vi "QuickDrop Populate QDKS Listbox.vi"(4 "Listbox Value":i32 caption="列表框值", 5 "Plugin Path":refnum<vi> caption="插件路径", 6 "Plugin Description String":refnum<vi> caption="插件说明字符串", 7 "QDKS Info":T1[](array[typedef]) caption="QDKS信息", 9 "Set Shortcut Boolean":refnum<vi> caption="设置快捷方式布尔", 10 "Shortcut String":refnum<vi> caption="快捷键字符串", 11 "Mappings Listbox":refnum<vi> caption="映射列表框") -> (0 "No Desc out":string="（无说明信息）" caption="无说明输出", 1 "Default out":string="%s（默认）" caption="默认输出", 2 "Control out":string="Ctrl-%s" caption="Ctrl组合输出")   [LabVIEW 2016]
uses:
  <resource>/dialog/QuickDrop/QuickDrop QDKS Info.ctl
panel:
  in  "No Desc":string="（无说明信息）" caption="无说明"
  in  "Control":string="Ctrl-%s" caption="Ctrl组合"
  in  "Default":string="%s（默认）" caption="默认"
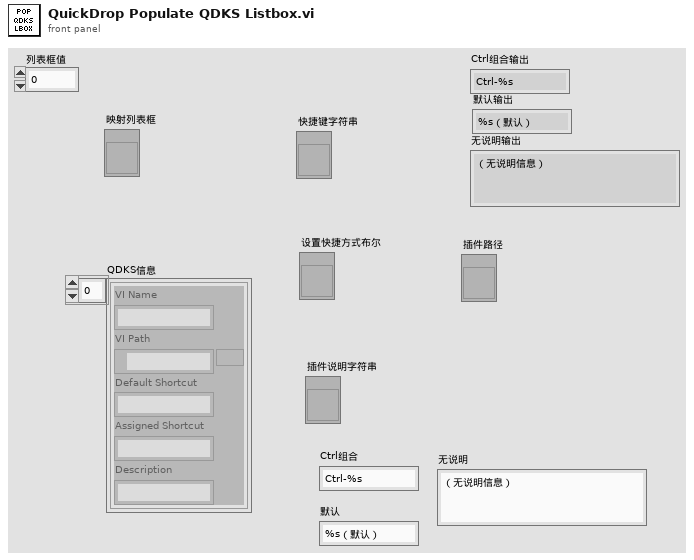
[diagram p1: front panel]
types:
  T1 = typedef "QuickDrop QDKS Info.ctl" = cluster{"VI Name":string, "VI Path":path, "Default Shortcut":string, "Assigned Shortcut":string, "Description":string}
  T2 = enum8{"Enabled", "Disabled", "Disabled and Grayed Out"}
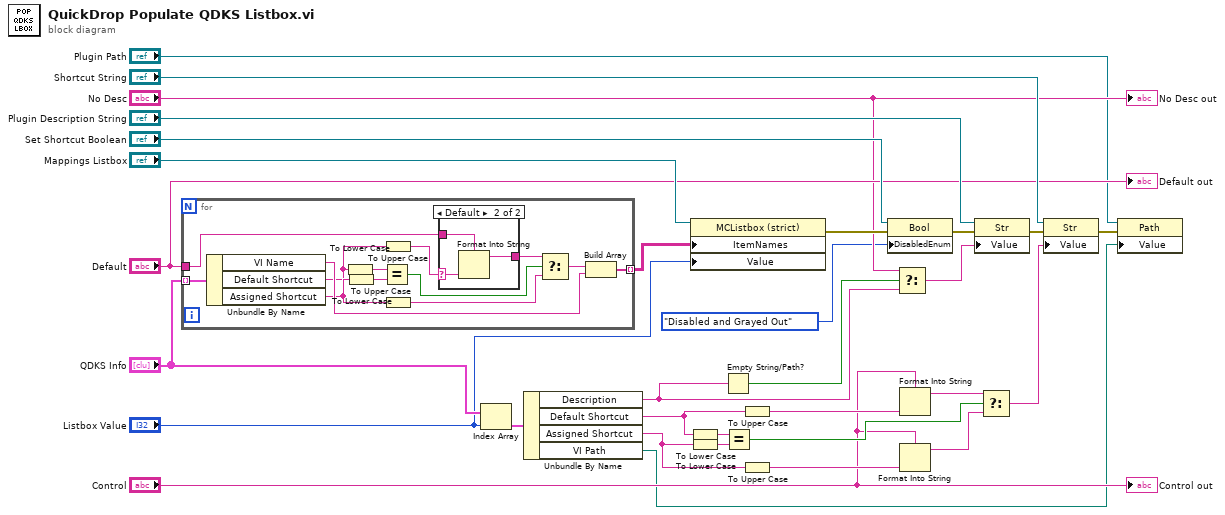
[diagram p0: block diagram]
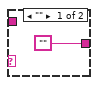
[diagram p2: hidden frame]
diagram:
  n1 = for {
    tunnel: "QDKS Info" -> [w44] mode=indexing
    tunnel: "Default" -> [w38]
    tunnel: [w32] -> w1 mode=indexing
    n2 = Unbundle By Name(w44) -> ("VI Name"=w43:string, "Default Shortcut"=w37:string, "Assigned Shortcut"=w41:string)
    n3 = To Lower Case(string=w37) -> (all lower case string=w34:string)
    n4 = To Lower Case(string=w41) -> (all lower case string=w33:string)
    n5 = Equal?(x=w34, y=w33) -> (x = y?=w42:bool)
    n6 = To Upper Case(1:w37) -> (0:w35:string)
    n7 = To Upper Case(1:w41) -> (0:w39:string)
    n8 = case shown="Default" w35 {
      selector: w35 -> [_ w46]
      tunnel: w38 -> [_ w48]
      tunnel: ["" w47] -> w36
      frame "" {
      }
      frame Default {
        n9 = Format Into String(format string=w48, w46) -> (resulting string=w47:string)  [unwired: 2 in, 1 out]
      }
    }
    n10 = Select(t=w36, s=w42, f=w39) -> (s? t:f=w40:string)
    n11 = Build Array(w40, w43) -> (w32:string[])
  }
  n12 = Index Array(array="QDKS Info", index="Listbox Value") -> (element=w25:T1)
  n13 = Unbundle By Name(w25) -> ("Description"=w14:string, "Default Shortcut"=w19:string, "Assigned Shortcut"=w23:string, "VI Path"=w2:path)
  n14 = To Lower Case(string=w19) -> (all lower case string=w7:string)
  n15 = To Lower Case(string=w23) -> (all lower case string=w6:string)
  n16 = property class="MCListbox (strict)"(reference="Mappings Listbox", "ItemNames"=w1, "Value"="Listbox Value") -> (error out=w30:errorcluster)  [unwired: 1 in, 1 out]
  n17 = Empty String/Path?(string/path=w14) -> (empty?=w15:bool)
  n18 = Equal?(x=w7, y=w6) -> (x = y?=w24:bool)
  n19 = To Upper Case(1:w19) -> (0:w17:string)
  n20 = To Upper Case(1:w23) -> (0:w10:string)
  n21 = property class="Bool"(reference="Set Shortcut Boolean", error in=w30, "DisabledEnum"=T2."Disabled and Grayed Out" ("Disabled")) -> (error out=w28:errorcluster)  [unwired: 1 out]
  n22 = Select(t="No Desc", s=w15, f=w14) -> (s? t:f=w12:string)
  n23 = Format Into String(format string="Control", w17) -> (resulting string=w18:string)  [unwired: 2 in, 1 out]
  n24 = Format Into String(format string="Control", w10) -> (resulting string=w9:string)  [unwired: 2 in, 1 out]
  n25 = property class="Str"(reference="Plugin Description String", error in=w28, "Value"=w12) -> (error out=w22:errorcluster)  [unwired: 1 out]
  n26 = Select(t=w18, s=w24, f=w9) -> (s? t:f=w20:string)
  n27 = property class="Str"(reference="Shortcut String", error in=w22, "Value"=w20) -> (error out=w4:errorcluster)  [unwired: 1 out]
  n28 = property class="Path"(reference="Plugin Path", error in=w4, "Value"=w2) -> ()  [unwired: 2 out]
  "Control out" <- "Control"
  "Default out" <- "Default"
  "No Desc out" <- "No Desc"
